vi "test_shitty.vi"() -> ()   [LabVIEW 2018]
panel:
  out "n_sync":i32[](array[numeric])
  out "count_channels 2":u32[](array[numeric])
  out "time_delays":i64[](array[numeric])
  out "count_timestamps":dbl[](array[numeric]) format="%#_12f"
  out "n_sync array":dbl[](array[numeric])
  out "channels":dbl[](array[numeric])
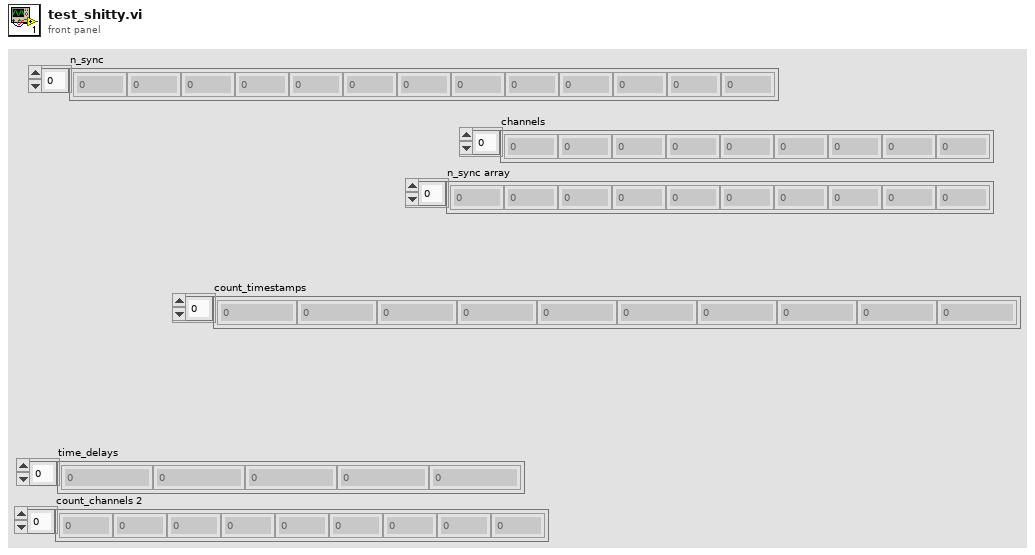
[diagram p1: front panel]
types:
  T1 = enum16{"big-endian, network order", "native, host order", "little-endian"}
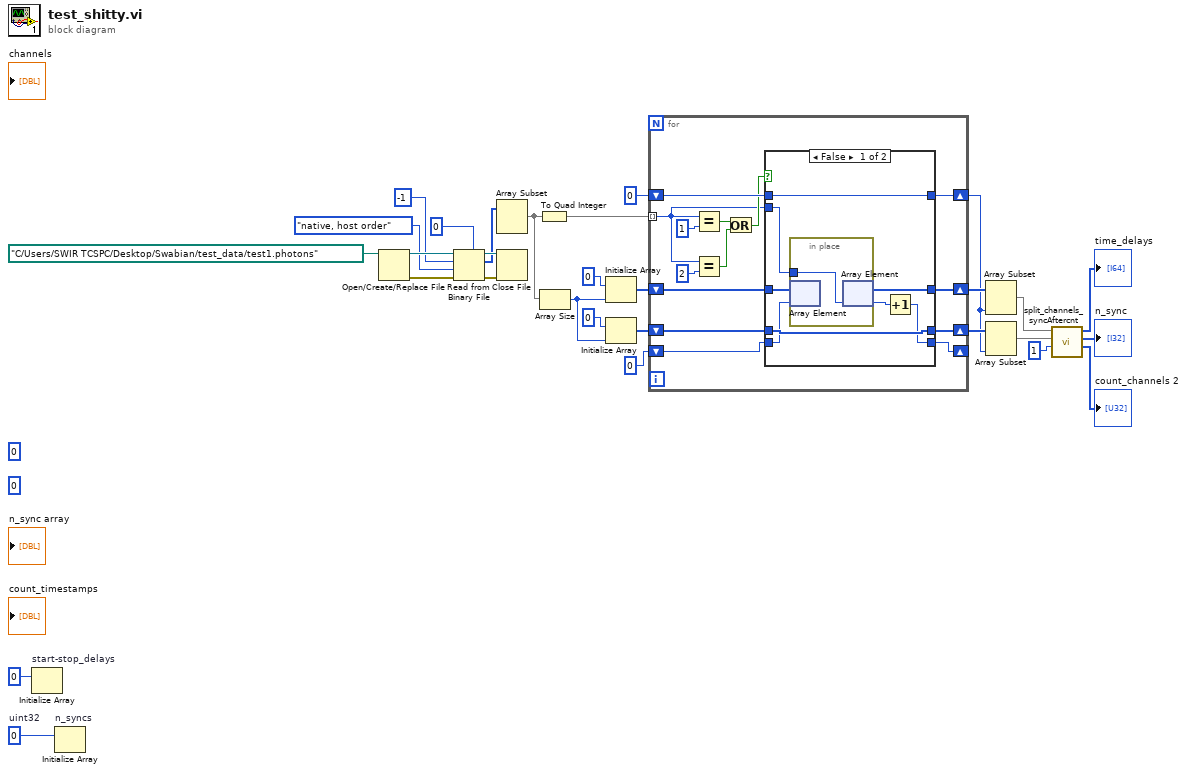
[diagram p0: block diagram]
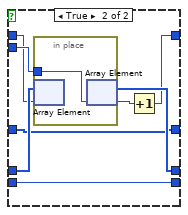
[diagram p2: hidden frame]
diagram:
  w9 = u32 0  # uint32
  (unwired) 0 ("element")
  (unwired) i64 0 ("element")
  n1 = Initialize Array "start-stop_delays"(i64 0 ("element")) -> ()  [unwired: 1 in, 1 out]
  n2 = Initialize Array "n_syncs"(w9) -> ()  [unwired: 1 in, 1 out]
  n3 = Open/Create/Replace File(file path (use dialog)=path "C:/Users/SWIR TCSPC/Desktop/Swabian/test_data/test1.photons") -> (refnum out=w28:refnum<file>, error out=w27:errorcluster)  [unwired: 5 in, 1 out]
  n4 = Read from Binary File(5:u64 0 ("element"), 8:w27, 9:T1."native, host order" ("byte order (0:big-endian, network order)"), 10:-1 ("count (1)"), 11:w28) -> (0:w24:errorcluster, 2:w5:u64[], 3:w25:refnum<file>)  [unwired: 1 in, 1 out]
  n5 = Array Subset(array=w5) -> (w4:u64[])  [unwired: 2 in]
  n6 = Close File(refnum=w25, error in=w24) -> ()  [unwired: 2 out]
  n7 = To Quad Integer(1:w4) -> (0:w14:i64[])
  n8 = Array Size(array=w4) -> (size(s)=w19:i32)
  n9 = Initialize Array(i64 0 ("element"), w19) -> (w16:i64[])
  n10 = Initialize Array(u32 0 ("element"), w19) -> (w18:u32[])
  n11 = for {
    tunnel: w14 -> [w36] mode=indexing
    shift-right: [w35] -> w13
    shift-left: w18 -> [w37]
    shift-right: [w34] -> w11
    shift-left: 0 ("element") -> [w39]
    shift-right: [w32] -> w12
    shift-left: w16 -> [w33]
    shift-right: [w30] -> _
    shift-left: 0 ("element") -> [w31]
    n12 = Equal?(x=w36, y=i64 1) -> (x = y?=w40:bool)
    n13 = Equal?(x=w36, y=i64 2) -> (x = y?=w41:bool)
    n14 = Or(x=w40, y=w41) -> (x .or. y?=w38:bool)
    n15 = case shown="False" w38 {
      tunnel: w39 -> [w51 w57]
      tunnel: w37 -> [w50 w60]
      tunnel: w36 -> [w44 w59]
      tunnel: [w50 w58] -> w35
      tunnel: [w51 w55] -> w34
      tunnel: w33 -> [w49 w53]
      tunnel: [w48 w53] -> w32
      tunnel: w31 -> [w47 w54]
      tunnel: [w45 w54] -> w30
      frame False {
        n16 = in-place {
          in-place-border: w44 -> [w52]
          n17 = in-place-array #1(w49, w47) -> ()  [unwired: 1 out]
          n18 = in-place-array #1(w52) -> (w48:i64[], w46:i32)
        }
        n19 = Increment(x=w46) -> (x+1=w45:i32)
      }
      frame True {
        n20 = in-place {
          in-place-border: w59 -> [w61]
          n21 = in-place-array #2(w60, w57) -> ()  [unwired: 1 out]
          n22 = in-place-array #2(w61) -> (w58:u32[], w56:i32)
        }
        n23 = Increment(x=w56) -> (x+1=w55:i32)
      }
    }
  }
  n24 = Array Subset(array=w12, length=w11) -> (w8:i64[])  [unwired: 1 in]
  n25 = Array Subset(array=w13, length=w11) -> (w7:u32[])  [unwired: 1 in]
  n26 = call "split_channels_syncAftercnt.vi"("sync_channel"=u32 1, "channels"=w7, "stamps"=w8) -> ("time_delays"=→"count_channels 2":i64[], "n_sync"=→"n_sync":i32[], "count_channels"=→"time_delays":u32[])  [unwired: 4 in, 2 out]
